vi "Add Records.vi"(8 "Error In (no error)":errorcluster, 10 "Expenses Tracker Records In":refnum<class "Expenses Tracker Record.lvclass">[](array[class]), 11 "SQLite DB Operator In":refnum<class "SQLite DB Operator.lvclass">) -> (0 "Error Out":errorcluster, 2 "Expenses Tracker Records Out":refnum<class "Expenses Tracker Record.lvclass">[](array[class]), 3 "SQLite DB Operator Out":refnum<class "SQLite DB Operator.lvclass">)   [LabVIEW 2023, in "SQLite DB Operator.lvclass"]
uses:
  SQLite DB Operator.lvclass
  SQLite DB Operator.lvclass/SQLite DB Operator.ctl
  <vilib>/drjdpowell/SQLite Library/SQL Connection/Connection.lvclass
  <vilib>/drjdpowell/SQLite Library/SQL Statement/SQL Statement.lvclass
  <vilib>/drjdpowell/SQLite Library/Transaction Helpers/Transaction.lvlib
  Private/VIs/Prepare Insert Command.vi
  DB Records/Expenses Tracker Record/Expenses Tracker Record.lvclass
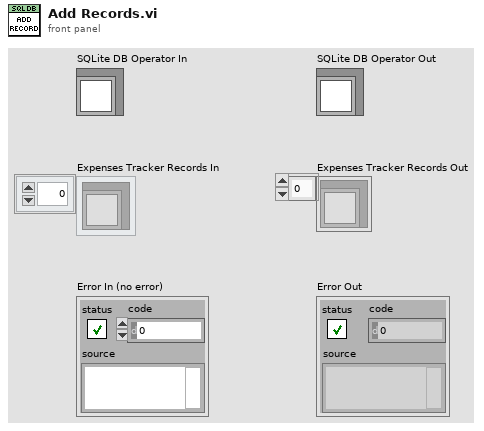
[diagram p1: front panel]
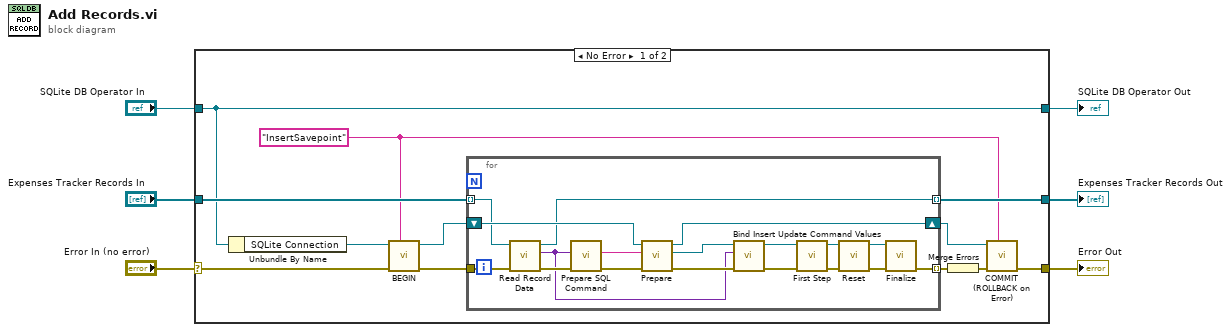
[diagram p0: block diagram]
diagram:
  n1 = case shown="No Error" "Error In (no error)" {
    selector: "Error In (no error)" -> [w16 w39]
    tunnel: [w10 w39] -> w4
    tunnel: [w17 w38] -> w6
    tunnel: "SQLite DB Operator In" -> [w17 w38]
    tunnel: "Expenses Tracker Records In" -> [w18 w37]
    tunnel: [w11 w37] -> w1
    frame No Error {
      w7 = "InsertSavepoint" ("Savepoint name")
      n2 = Unbundle By Name(w17) -> ("SQLite Connection"=w14:refnum<class "Connection.lvclass">)
      n3 = call <vilib>:"BEGIN.vi"("Savepoint name"=w7, "error in (no error)"=w16, "SQLite Connection in"=w14) -> ("error out"=w15:errorcluster, "SQLite Connection"=w13:refnum<class "Connection.lvclass">)  [unwired: 7 in]
      n4 = for {
        tunnel: w15 -> [w36]
        tunnel: w18 -> [w20] mode=indexing
        tunnel: [w31] -> w12 mode=indexing
        tunnel: [w19] -> w11 mode=indexing
        shift-right: [w24] -> w8
        shift-left: w13 -> [w27]
        n5 = call-dynamic "Read Record Data.vi"("Error In (no error)"=w36, "Expenses Tracker Record In"=w20) -> ("Error Out"=w30:errorcluster, "Record"=w22:variant, "Expenses Tracker Record Out"=w19:refnum<class "Expenses Tracker Record.lvclass">)  [unwired: 7 in]
        n6 = call-poly "Prepare SQL Command.vi"("Error In (no error)"=w30, "Record"=w22) -> ("Error Out"=w25:errorcluster, "Insert SQL Command"=w21:string)  [unwired: 8 in]
        n7 = call <vilib>:"Prepare.vi"("error in (no error)"=w25, "SQL"=w21, "SQLite Connection in"=w27) -> ("error out"=w23:errorcluster, "SQL Statement"=w26:refnum<class "SQL Statement.lvclass">, "SQLite Connection"=w24:refnum<class "Connection.lvclass">)  [unwired: 4 in, 2 out]
        n8 = call "Bind Insert Update Command Values.vi"("Error In (no error)"=w23, "Record"=w22, "SQL Statement In"=w26) -> ("Error Out"=w28:errorcluster, "SQL Statement Out"=w29:refnum<class "SQL Statement.lvclass">)  [unwired: 7 in]
        n9 = call <vilib>:"First Step.vi"("error in (no error)"=w28, "SQL Statement in"=w29) -> ("error out"=w33:errorcluster, "SQL Statement"=w32:refnum<class "SQL Statement.lvclass">)  [unwired: 7 in, 1 out]
        n10 = call <vilib>:"Reset.vi"("error in (no error)"=w33, "SQL Statement in"=w32) -> ("error out"=w35:errorcluster, "SQL Statement"=w34:refnum<class "SQL Statement.lvclass">)  [unwired: 8 in]
        n11 = call <vilib>:"Finalize.vi"("error in (no error)"=w35, "SQL Statement in"=w34) -> ("error out"=w31:errorcluster)  [unwired: 9 in]
      }
      n12 = Merge Errors(w12) -> (w9:errorcluster)
      n13 = call <vilib>:"COMMIT (ROLLBACK on Error).vi"("Savepoint name"=w7, "error in (no error)"=w9, "SQLite Connection in"=w8) -> ("error out"=w10:errorcluster)  [unwired: 7 in, 1 out]
    }
    frame Error {
    }
  }
  "Error Out" <- w4
  "SQLite DB Operator Out" <- w6
  "Expenses Tracker Records Out" <- w1
